vi "Write Elastic Moduli Configuration.vi"(8 "error in (no error)":errorcluster, 10 "Elastic Moduli Configuration":T1={"Output header "="", "rusin\n.dat"=enum."NONE", "Resonance detector module name"="", "Save sp*.dat"=TRUE}, 11 "Elastic Moduli in":refnum<class "Format Resonances.lvclass">) -> (0 "error out":errorcluster, 3 "Elastic Moduli out":refnum<class "Format Resonances.lvclass">)   [LabVIEW 2019, in "Format Resonances.lvclass"]
uses:
  Format Resonances.lvclass
  C:/GitHub/LabActor/Template Module/Template Module.lvclass
  Format Resonances Configuration.ctl
  Template Module/Template Module.lvclass/Template Module.ctl
  Template Module/Write Configuration.vi
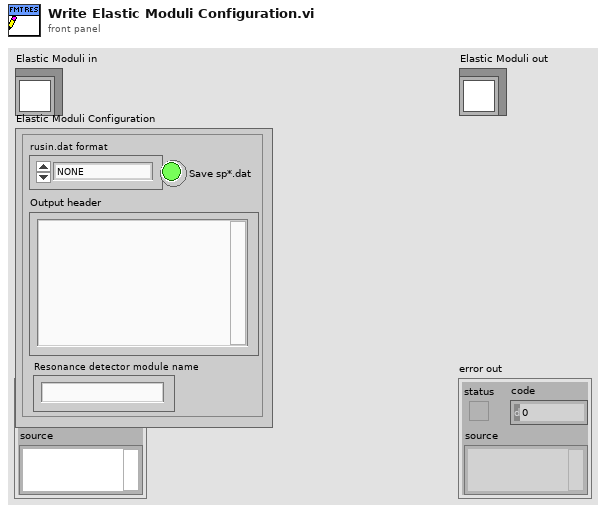
[diagram p1: front panel]
types:
  T1 = typedef "Format Resonances Configuration.ctl" = cluster{"Output header ":string, "rusin\n.dat":enum16{"NONE", "With header", "Without header"}, "Resonance detector module name":string, "Save sp*.dat":bool}
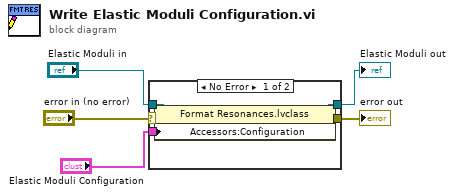
[diagram p0: block diagram]
diagram:
  n1 = case shown="No Error" "error in (no error)" {
    selector: "error in (no error)" -> [w7 w11]
    tunnel: [w6 w11] -> w4
    tunnel: [w8 w12] -> w2
    tunnel: "Elastic Moduli in" -> [w10 w12]
    tunnel: "Elastic Moduli Configuration" -> [w9 _]
    frame No Error {
      n2 = property class="Format Resonances.lvclass"(reference=w10, error in=w7, "Accessors:Configuration"=w9) -> (reference out=w8:refnum<class "Format Resonances.lvclass">, error out=w6:errorcluster)
    }
    frame Error {
    }
  }
  "error out" <- w4
  "Elastic Moduli out" <- w2
